vi "Open Subpanel UI Reference.vi"(0 "Plugin in":refnum<class "Generic Plugin.lvclass">, 1 "error in (no error)":errorcluster) -> (2 "Plugin out":refnum<class "Generic Plugin.lvclass">, 3 "vi reference":refnum<vi>, 4 "error out":errorcluster)   [LabVIEW 2020, in "RxnRover.lvlib" / "Generic Plugin.lvclass"]
doc: "Get a reference for the Subpanel UI.vi of the controller."
uses:
  Generic Plugin.lvclass
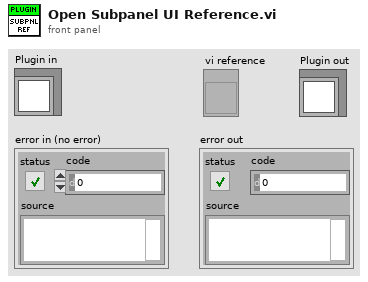
[diagram p1: front panel]
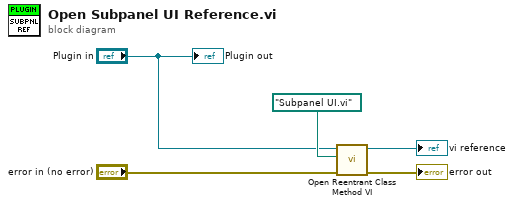
[diagram p0: block diagram]
diagram:
  n1 = call "Open Reentrant Class Method VI.vi"("error in (no error)"="error in (no error)", "Method VI Filename to Open"=path "Subpanel UI.vi" ("name or relative path"), "Generic Plugin in"="Plugin in") -> ("error out"=→"error out":errorcluster, "VI Refnum"=→"vi reference":refnum<vi>)  [unwired: 7 in]
  "Plugin out" <- "Plugin in"
